vi "Cycle.vi"(8 "error in (no error)":errorcluster, 11 "MouseDotMapping In":refnum<class "MouseDotMapping.lvclass">) -> (0 "error out":errorcluster, 3 "MouseDotMapping Out":refnum<class "MouseDotMapping.lvclass">)   [LabVIEW 2014, in "MouseDotMapping.lvclass"]
uses:
  MouseDotMapping.lvclass
  Trial Based Experiment Statechart/PassiveExperiment/PassiveExperiment.lvclass
panel:
  out "ExperimentStats":T1
  in  "FixationRadius 2":dbl=34.0
  in  "RewardAmount 2":dbl=50.0
  out "Timeouts":T2={"Intertrial"=1500.0, "AcquireFixation"=4000.0, "HoldFixation"=300.0, "DelayPeriod"=2000.0, "ResponsePeriod"=0.0}
  in  "Eye Params 2":dbl[](array[numeric])
  out "XY Graph 2":cluster{"horizontal":dbl[], "vertical":dbl[]}[](graph)
  out "Elapsed Time (s)":dbl
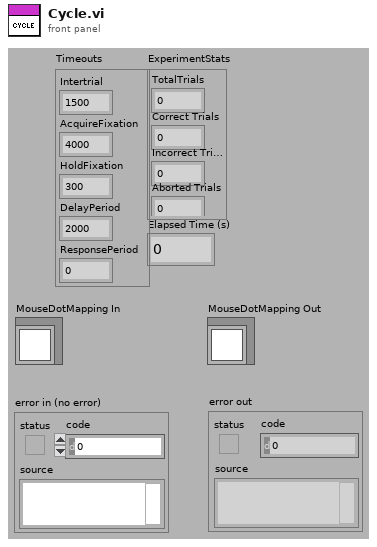
[diagram p1: front panel]
types:
  T1 = cluster{"TotalTrials":dbl, "Correct Trials":dbl, "Incorrect Trials":dbl, "Aborted Trials":dbl}
  T2 = cluster{"Intertrial":dbl, "AcquireFixation":dbl, "HoldFixation":dbl, "DelayPeriod":dbl, "ResponsePeriod":dbl}
  T3 = cluster{"TotalTrials":u32, "Correct Trials":u32, "Incorrect Trials":u32, "Aborted Trials":u32}
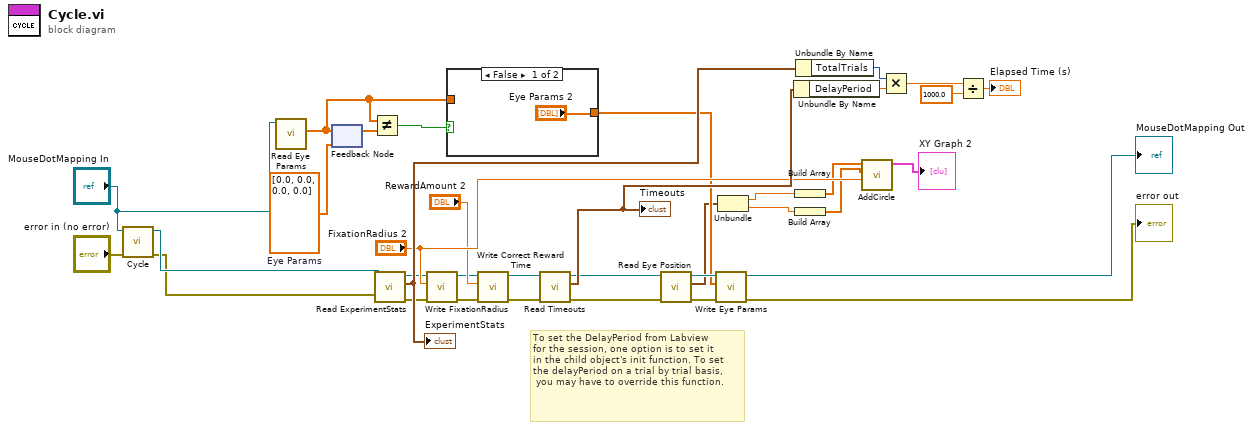
[diagram p0: block diagram]
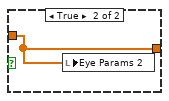
[diagram p2: hidden frame]
diagram:
  w11 = dbl[] [0.0, 0.0, 0.0, 0.0]  # Eye Params
  # "To set the DelayPeriod from Labview\nfor the session, one option is to set it \nin the child object's init function. To set\nthe delayPeriod on a trial by trial basis,\n you may have to override this function."
  n1 = call-parent "Cycle.vi"("error in (no error)"="error in (no error)", "PassiveExperiment In"="MouseDotMapping In") -> ("error out"=w1:errorcluster, "PassiveExperiment Out"=w2:refnum<class "MouseDotMapping.lvclass">)  [unwired: 8 in]
  n2 = call-dynamic "Read Eye Params.vi"("TrialBasedExperiment in"="MouseDotMapping In") -> ("Eye Params"=w10:dbl[])  [unwired: 8 in, 2 out]
  n3 = feedback #1(w11) -> (w13:dbl[])
  n4 = feedback-in #1(w10) -> ()
  n5 = Not Equal?(x=w10, y=w13) -> (x != y?=w12:bool)
  n6 = call-dynamic "Read ExperimentStats.vi"("error in (no error)"=w1, "TrialBasedExperiment in"=w2) -> ("error out"=w20:errorcluster, "ExperimentStats"=w34:T3, "TrialBasedExperiment out"=w21:refnum<class "MouseDotMapping.lvclass">)  [unwired: 7 in]
  "ExperimentStats" <- w34
  n7 = call-dynamic "Write FixationRadius.vi"("error in (no error)"=w20, "FixationRadius"="FixationRadius 2", "MatlabExperiment in"=w21) -> ("error out"=w17:errorcluster, "MatlabExperiment out"=w18:refnum<class "MouseDotMapping.lvclass">)  [unwired: 7 in]
  n8 = case shown="False" w12 {
    tunnel: ["Eye Params 2" w38] -> w7
    tunnel: w10 -> [_ w38]
    frame False {
    }
    frame True {
      n9 = local write "Eye Params 2"(w38) -> ()
    }
  }
  n10 = call-dynamic "Write Correct Reward Time.vi"("error in (no error)"=w17, "Correct Reward Time"="RewardAmount 2", "MatlabExperiment in"=w18) -> ("error out"=w15:errorcluster, "MatlabExperiment out"=w16:refnum<class "MouseDotMapping.lvclass">)  [unwired: 7 in]
  n11 = call-dynamic "Read Timeouts.vi"("error in (no error)"=w15, "TrialBasedExperiment in"=w16) -> ("error out"=w14:errorcluster, "Timeouts"=w35:T2, "TrialBasedExperiment out"=w28:refnum<class "MouseDotMapping.lvclass">)  [unwired: 7 in]
  "Timeouts" <- w35
  n12 = call-dynamic "Read Eye Position.vi"("error in (no error)"=w14, "TrialBasedExperiment in"=w28) -> ("error out"=w8:errorcluster, "Eye Position"=w6:cluster{"Horizontal":dbl, "Vertical":dbl}, "TrialBasedExperiment out"=w9:refnum<class "MouseDotMapping.lvclass">)  [unwired: 7 in]
  n13 = call-dynamic "Write Eye Params.vi"("error in (no error)"=w8, "Eye Params"=w7, "TrialBasedExperiment in"=w9) -> ("error out"=→"error out":errorcluster, "TrialBasedExperiment out"=→"MouseDotMapping Out":refnum<class "MouseDotMapping.lvclass">)  [unwired: 7 in]
  n14 = Unbundle(w6) -> ("Horizontal"=w22:dbl, "Vertical"=w23:dbl)
  n15 = Unbundle By Name(w35) -> ("DelayPeriod"=w32:dbl)
  n16 = Build Array(w22) -> (w24:dbl[])
  n17 = Build Array(w23) -> (w25:dbl[])
  n18 = Unbundle By Name(w34) -> ("TotalTrials"=w31:u32)
  n19 = call "AddCircle.vi"("radius"="FixationRadius 2", "vertical"=w25, "horizontal"=w24) -> ("output"=→"XY Graph 2":cluster{"horizontal":dbl[], "vertical":dbl[]}[])  [unwired: 8 in]
  n20 = Multiply(x=w31, y=w32) -> (x*y=w29:dbl)
  n21 = Divide(x=w29, y=1000.0) -> (x/y=→"Elapsed Time (s)":dbl)
